vi "from string.vi"(8 "error in":errorcluster, 9 "data":string, 10 "version":string, 11 "configuration in":refnum<class "NISE_CEF_serializable configuration.lvclass">) -> (0 "error out":errorcluster, 3 "configuration out":refnum<class "NISE_CEF_serializable configuration.lvclass">)   [LabVIEW 2013, in "NISE_CEF_serializable configuration.lvclass"]
doc: "Provides an interface for loading a module configuration from a file or other serialized data source. It is recommended that all children of this class store data in two sets--data required for its own initialization, and any data required for parent initialization--and that each implementation uses the <b>Call Parent Method</b> primitive to de-serialize parent information."
uses:
  NISE_CEF_serializable configuration.lvclass
  NISE_CEF_serializable configuration.lvclass/NISE_CEF_serializable configuration.ctl
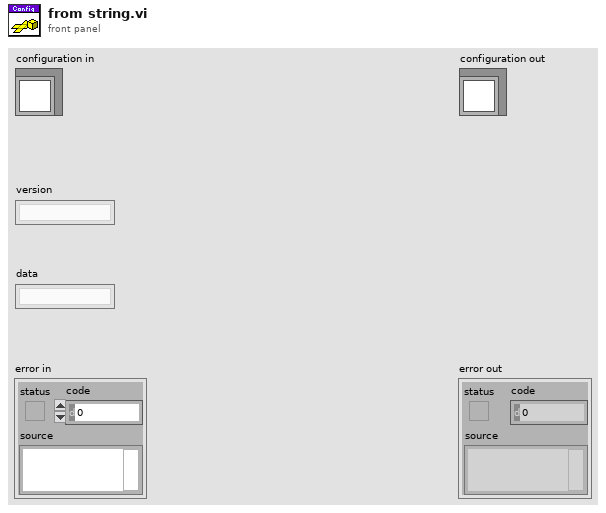
[diagram p1: front panel]
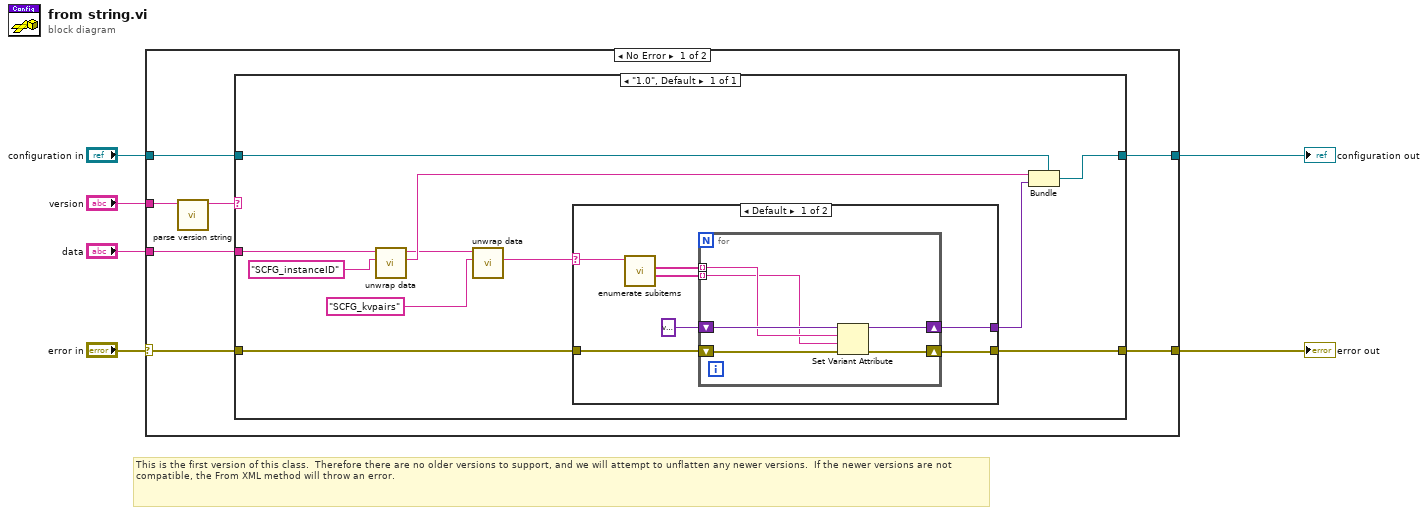
[diagram p0: block diagram]
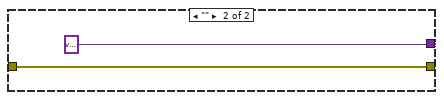
[diagram p2: hidden frame]
diagram:
  # "This is the first version of this class.  Therefore there are no older versions to support, and we will attempt to unflatten any newer versions.  If the newer versions are not compatible, the From XML method will throw an error."
  n1 = case shown="No Error" "error in" {
    selector: "error in" -> [w8 w41]
    tunnel: "data" -> [w13 _]
    tunnel: "configuration in" -> [w12 w40]
    tunnel: [w11 w40] -> w1
    tunnel: [w7 w41] -> w2
    tunnel: "version" -> [w10 _]
    frame No Error {
      n2 = call "parse version string.vi"("full version"=w10) -> ("major.minor version"=w9:string)  [unwired: 7 in, 3 out]
      n3 = case shown="\"1.0\", Default" w9 {
        tunnel: w13 -> [w22]
        tunnel: w8 -> [w17]
        tunnel: w12 -> [w24]
        tunnel: [w23] -> w11
        tunnel: [w14] -> w7
        frame "1.0", Default {
          n4 = call "unwrap data.vi"("identifier"="SCFG_instanceID" ("additional identifier"), "data to unwrap"=w22) -> ("unwrapped data"=w20:string, "remaining string"=w19:string)  [unwired: 8 in]
          n5 = call "unwrap data.vi"("identifier"="SCFG_kvpairs" ("additional identifier"), "data to unwrap"=w19) -> ("unwrapped data"=w16:string)  [unwired: 8 in, 1 out]
          n6 = case shown="Default" w16 {
            selector: w16 -> [w28 _]
            tunnel: w17 -> [w27 w38]
            tunnel: [w30 variant ("key-value pairs")] -> w15
            tunnel: [w29 w38] -> w14
            frame Default {
              n7 = call "enumerate subitems.vi"("data to enumerate"=w28) -> ("associated data"=w25:string[], "discovered subitems"=w26:string[])  [unwired: 8 in, 1 out]
              n8 = for {
                shift-right: [w36] -> w30
                shift-left: variant ("key-value pairs") -> [w37]
                shift-right: [w34] -> w29
                shift-left: w27 -> [w35]
                tunnel: w26 -> [w33] mode=indexing
                tunnel: w25 -> [w32] mode=indexing
                n9 = Set Variant Attribute(Variant=w37, name=w33, value=w32, error in=w35) -> (Variant out=w36:variant, error out=w34:errorcluster)  [unwired: 1 out]
              }
            }
            frame "" {
            }
          }
          n10 = Bundle(cluster=w24, w20, w15) -> (w23:refnum<class "NISE_CEF_serializable configuration.lvclass">)
        }
      }
    }
    frame Error {
    }
  }
  "error out" <- w2
  "configuration out" <- w1
